vi "libssh2_session_methods.vi"(8 "error in (no error)":errorcluster, 10 "method_type":T1, 11 "session":T2) -> (0 "error out":errorcluster, 2 "methods":string)   [LabVIEW 2013, in "libssh2.lvlib"]
doc: "Get the methods negotiated for a session."
uses:
  libssh2.lvlib
  Session Refnum.ctl
  libssh2_method_type.ctl
  Not A Session.vi
  <vilib>/Utility/error.llb/Error Cluster From Error Code.vi
  Global Settings.vi
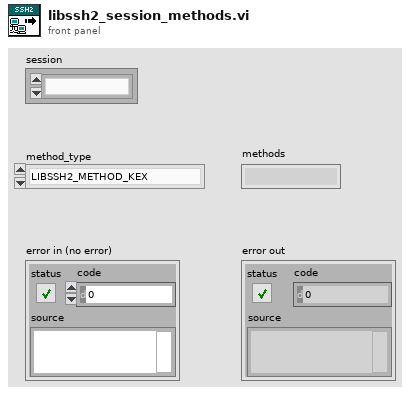
[diagram p1: front panel]
types:
  T1 = typedef "libssh2.lvlib/libssh2_method_type.ctl" = enum16{"LIBSSH2_METHOD_KEX", "LIBSSH2_METHOD_HOSTKEY", "LIBSSH2_METHOD_CRYPT_CS", "LIBSSH2_METHOD_CRYPT_SC", "LIBSSH2_METHOD_MAC_CS", "LIBSSH2_METHOD_MAC_SC", "LIBSSH2_METHOD_COMP_CS", "LIBSSH2_METHOD_COMP_SC", "LIBSSH2_METHOD_LANG_CS", "LIBSSH2_METHOD_LANG_SC", "LIBSSH2_METHOD_SIGN_ALGO"}
  T2 = typedef "libssh2.lvlib/Session Refnum.ctl" = refnum<k1>
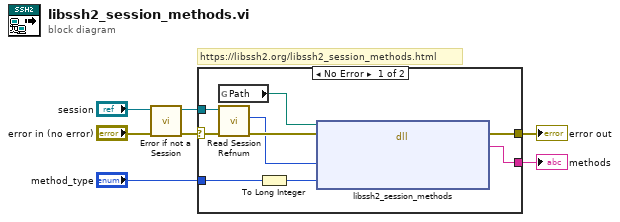
[diagram p0: block diagram]
diagram:
  # "https://libssh2.org/libssh2_session_methods.html"
  n1 = call "Error if not a Session.vi"("error in (no error)"="error in (no error)", "session"="session") -> ("error out"=w5:errorcluster, "session out"=w3:T2)  [unwired: 8 in]
  n2 = case shown="No Error" w5 {
    selector: w5 -> [w15 w17]
    tunnel: [w16 w17] -> w7
    tunnel: w3 -> [w14 _]
    tunnel: [w8 _] -> w2
    tunnel: "method_type" -> [w10 _]
    frame No Error {
      n3 = global read "Global Settings.vi" "Path"() -> (w11:path)
      n4 = call "Read Session Refnum.vi"("error in (no error)"=w15, "session"=w14) -> ("error out"=w13:errorcluster, "LIBSSH2_SESSION*"=w12:u64)  [unwired: 5 in, 3 out]
      n5 = To Long Integer(number=w10) -> (32bit integer=w9:i32)
      n6 = dll-call lib="?" fn="libssh2_session_methods"(path in=w11, error in=w13, "session"=w12, "method_type"=w9) -> (error out=w16:errorcluster, "return value"=w8:string)  [unwired: 3 in, 1 out]
    }
    frame Error {
    }
  }
  "error out" <- w7
  "methods" <- w2
